vi "Copy Template.vi"(8 "error in":errorcluster, 11 "Destination Directory":path) -> (0 "error out":errorcluster, 3 "new path":path)   [LabVIEW 2017]
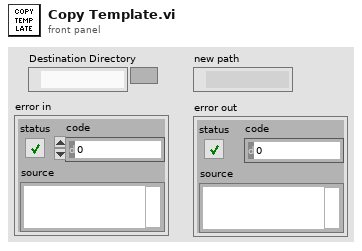
[diagram p1: front panel]
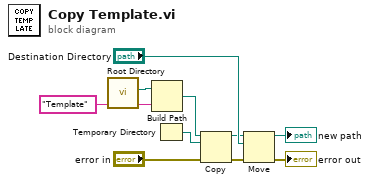
[diagram p0: block diagram]
diagram:
  n1 = call "Root Directory.vi"() -> ("root directory"=w5:path)  [unwired: 11 in]
  n2 = Build Path(base path=w5, name or relative path="Template") -> (appended path=w7:path)
  n3 = Temporary Directory() -> (w10:path)
  n4 = Copy(8:"error in", 10:w10, 11:w7) -> (0:w3:errorcluster, 3:w8:path)  [unwired: 2 in, 1 out]
  n5 = Move(source path=w8, error in=w3, 10:"Destination Directory") -> (error out=→"error out":errorcluster, 3:→"new path":path)  [unwired: 2 in, 1 out]
